vi "patchcontrol.vi"() -> ()   [LabVIEW 2010]
uses:
  <vilib>/DAQmx/write.llb/DAQmx Write (Analog Wfm 1Chan NSamp).vi
  <vilib>/DAQmx/create/channels.llb/DAQmx Create Channel (AO-Voltage-Basic).vi
  <vilib>/DAQmx/configure/timing.llb/DAQmx Timing (Use Waveform).vi
  <vilib>/daqmx/miscellaneous.llb/DAQmx Fill In Error Info.vi
  <vilib>/measure/NI_MABase.lvlib
  Program Files/National Instruments/LabVIEW 2010/resource/objmgr/daqmx.rc
panel:
  in  "stop":bool
  out "Waveform Graph":waveform(dbl)(graph)={"t0"=timestamp(1226.0 s since 1904-01-01), "dt"=0.001, "Y"=array[1000 elements]}
  in  "duty cycle (%)":dbl=50.0
  in  "sampling info":cluster{"Fs":dbl, "#s":dbl}={"Fs"=1000.0, "#s"=1000.0}
  in  "phase":dbl
  in  "amplitude":dbl=0.1
  in  "frequency":dbl=100.0
  in  "offset":dbl
  in  "Enum":enum16{"Seal test", "square wave", ""}(ring)=enum."square wave"
  in  "Voltage":tag="Dev1/ao2"
  in  "AO.DataXferReqCond":i32(ring)=10235 items=["Onboard Memory Empty"=10235, "Onboard Memory Half Full or Less"=10239, "Onboard Memory Less than Full"=10242]
  in  "AO.DataXferMech":i32(ring)=10054 items=["DMA"=10054, "Interrupts"=10204, "Programmed I/O"=10264, "USB Bulk"=12590]
  in  "AO.TermCfg":i32(ring)=10083 items=["RSE"=10083, "Differential"=10106, "Pseudodifferential"=12529]
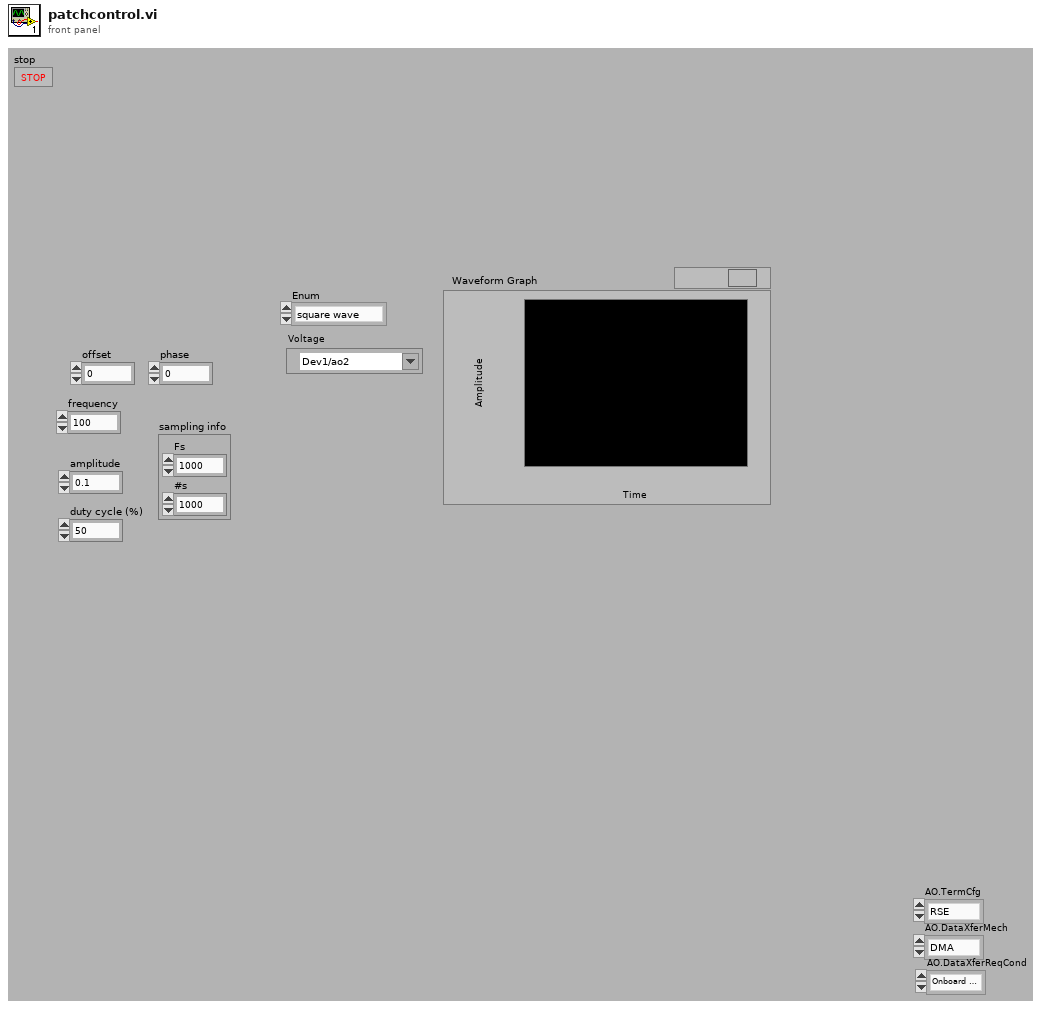
[diagram p1: front panel]
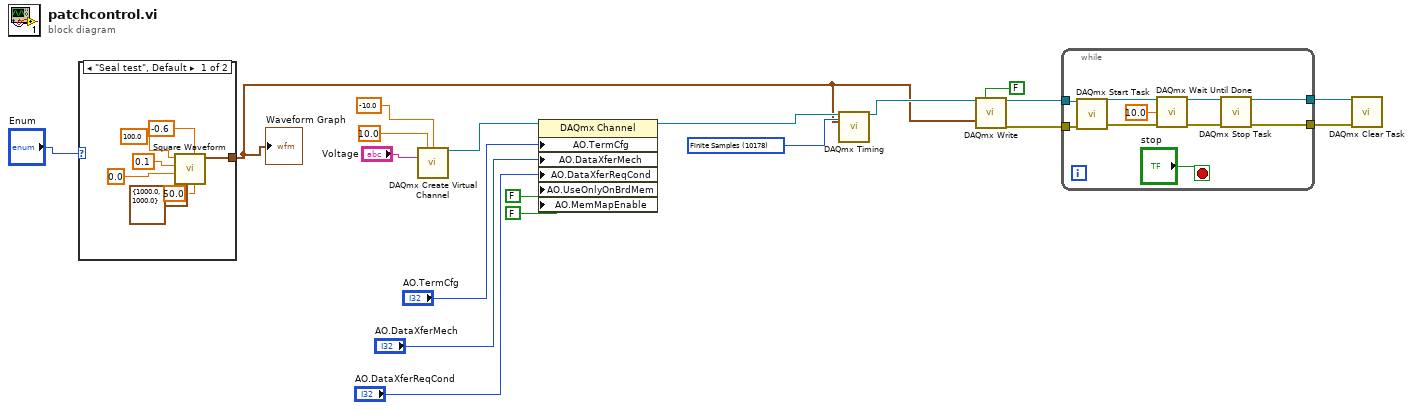
[diagram p0: block diagram]
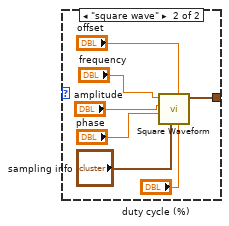
[diagram p2: hidden frame]
diagram:
  w16 = 10178 items=["Finite Samples"=10178, "Continuous Samples"=10123, "Hardware Timed Single Point"=12522] ("sample mode")
  n1 = case shown="\"Seal test\", Default" "Enum" {
    tunnel: [w20 w27] -> w4
    frame "Seal test", Default {
      n2 = call <vilib>:"Square Waveform.vi"("duty cycle (%)"=50.0, "offset"=-0.6, "sampling info"=cluster{"Fs":dbl, "#s":dbl} {"Fs"=1000.0, "#s"=1000.0}, "phase"=0.0, "amplitude"=0.1, "frequency"=100.0) -> ("signal out"=w20:waveform(dbl))  [unwired: 4 in, 1 out]
    }
    frame "square wave" {
      n3 = call <vilib>:"Square Waveform.vi"("duty cycle (%)"="duty cycle (%)", "offset"="offset", "sampling info"="sampling info", "phase"="phase", "amplitude"="amplitude", "frequency"="frequency") -> ("signal out"=w27:waveform(dbl))  [unwired: 4 in, 1 out]
    }
  }
  "Waveform Graph" <- w4
  n4 = call-poly <vilib>:"DAQmx Create Virtual Channel.vi"("maximum value"=10.0, "minimum value"=-10.0, "physical channels"="Voltage") -> ("task out"=w7:refnum<k21>)  [unwired: 6 in, 6 out]
  n5 = property class="DAQmx Channel"(reference=w7, "AO.TermCfg"="AO.TermCfg", "AO.DataXferMech"="AO.DataXferMech", "AO.DataXferReqCond"="AO.DataXferReqCond", "AO.UseOnlyOnBrdMem"=FALSE, "AO.MemMapEnable"=FALSE) -> (reference out=w15:refnum<k21>)  [unwired: 1 in, 1 out]
  n6 = call-poly <vilib>:"DAQmx Timing.vi"("task/channels in"=w15, "sample mode"=w16, "waveform"=w4) -> ("task out"=w19:refnum<k21>)  [unwired: 2 in, 10 out]
  n7 = call-poly <vilib>:"DAQmx Write.vi"("task/channels in"=w19, "auto start"=FALSE, "data"=w4) -> ("task out"=w17:refnum<k21>, "error out"=w3:errorcluster)  [unwired: 1 in, 10 out]
  n8 = while {
    tunnel: w17 -> [w43]
    tunnel: w3 -> [w42]
    tunnel: [w36] -> w2
    tunnel: [w34] -> w1
    stop <- "stop" stop-if-true
    n9 = call <vilib>:"DAQmx Start Task.vi"("task/channels in"=w43, "error in"=w42) -> ("task out"=w41:refnum<k21>, "error out"=w40:errorcluster)  [unwired: 12 out]
    n10 = call <vilib>:"DAQmx Wait Until Done.vi"("task/channels in"=w41, "timeout (sec)"=10.0, "error in"=w40) -> ("task out"=w37:refnum<k21>, "error out"=w35:errorcluster)  [unwired: 11 in]
    n11 = call <vilib>:"DAQmx Stop Task.vi"("task/channels in"=w37, "error in"=w35) -> ("task out"=w36:refnum<k21>, "error out"=w34:errorcluster)  [unwired: 12 in]
  }
  n12 = call <vilib>:"DAQmx Clear Task.vi"("task in"=w2, "error in"=w1) -> ()  [unwired: 14 out]
